vi "simple Calibration.vi"() -> ()   [LabVIEW 2020]
uses:
  <vilib>/vision/NI_Vision_Development_Module.lvlib
panel:
  out "Number of Particles":i32
  in  "stop":bool
  out "Image":T1(plugin-control)
  out "error out":errorcluster
  out "Distanza punto iniziale-finale [mm]":sgl[](array[numeric]) format="%.2f"
  in  "P1":i32
  in  "P0":i32
  in  "error in":errorcluster
  in  "Input Image Path":path=path "C:/Users/Dell/Desktop/Esame/LOAD/SimpleCalibration/CalibGrid2_Crop.png"
  out "Image":T1(plugin-control)
  in  "Risoluzione Spaziale":T2={"X Step"=1.0, "Y Step"=1.0, "Unit"=enum."Undefined"} {"Y Step" format="%.2f"; "X Step" format="%.2f"}
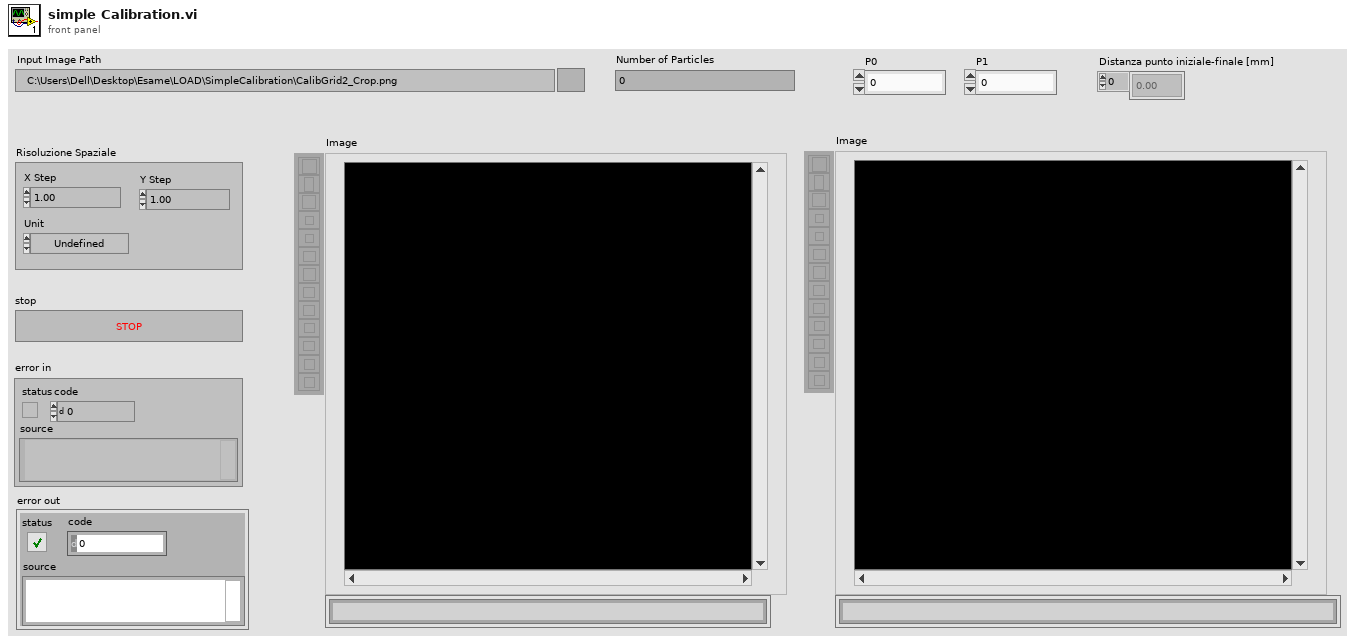
[diagram p1: front panel]
types:
  T1 = typedef "IMAQ Image.ctl" = refnum<image>
  T2 = typedef "Simple Grid Descriptor" = cluster{"X Step":sgl, "Y Step":sgl, "Unit":T3}
  T3 = typedef "Image Unit" = enum32{"Undefined", "Angström", "Micrometer", "Millimeter", "Centimeter", "Meter", "Kilometer", "Microinch", "Inch", "Feet", "Nautical miles", "Standard miles", "Steps"}
  T4 = cluster{"Area":dbl, "Number of Holes":dbl, "Bounding Rect":cluster{"Left":dbl, "Top":dbl, "Right":dbl, "Bottom":dbl}, "Center of Mass":cluster{"X":dbl, "Y":dbl}, "Orientation":dbl, "Dimensions":cluster{"Width":dbl, "Height":dbl}}[]
  T5 = cluster{"Desired Font (Application)":enum16{"User-specified Font", "Application Font", "System Font", "Dialog Font"}, "[User-specified Font]":cluster{"Font Name":string, "Size":i16, "Strikeout?":bool, "Italic?":bool, "Underline?":bool, "Outline?":bool, "Shadow?":bool, "Bold?":bool, "Rotation Angle":dbl}, "Horizontal Alignment":i16, "Vertical Alignment":i16}
  T6 = cluster{"Left":dbl, "Top":dbl, "Right":dbl, "Bottom":dbl}
  T7 = cluster{"Area":dbl, "Number of Holes":dbl, "Bounding Rect":cluster{"Left":dbl, "Top":dbl, "Right":dbl, "Bottom":dbl}, "Center of Mass":cluster{"X":dbl, "Y":dbl}, "Orientation":dbl, "Dimensions":cluster{"Width":dbl, "Height":dbl}}
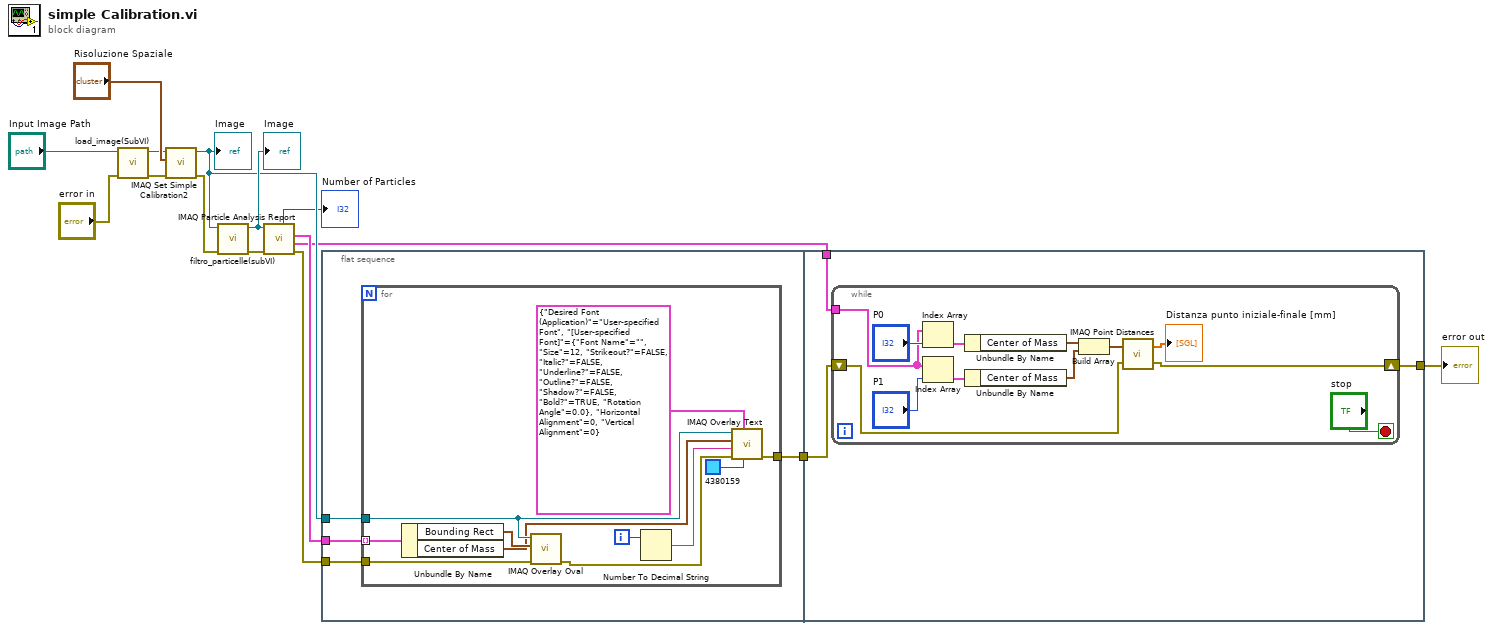
[diagram p0: block diagram]
diagram:
  n1 = call "load_image(SubVI).vi"("error in (no error)"="error in", "Image Path"="Input Image Path") -> ("error out"=w11:errorcluster, "Image GRAY"=w12:T1)  [unwired: 8 in]
  n2 = call "IMAQ Set Simple Calibration2"("error in (no error)"=w11, "Pixel Distances"="Risoluzione Spaziale", "Image"=w12) -> ("error out"=w10:errorcluster, "Calibration Template Image"=w6:T1)  [unwired: 7 in]
  "Image" <- w6
  n3 = call "filtro_particelle(subVI).vi"("error in (no error)"=w10, "Image Src"=w6) -> ("error out"=w8:errorcluster, "Image"=w9:T1)  [unwired: 8 in]
  "Image" <- w9
  n4 = call "IMAQ Particle Analysis Report"("error in (no error)"=w8, "Image"=w9) -> ("error out"=w7:errorcluster, "Particle Reports (Real-World)"=w2:T4, "Particle Reports (Pixels)"=w5:T4, "Number of Particles"=→"Number of Particles":i32)  [unwired: 4 in, 2 out]
  n5 = flat-sequence {
    tunnel: w7 -> [w19]
    tunnel: w6 -> [w18]
    tunnel: w5 -> [w17]
    tunnel: [w16] -> w3
    tunnel: [w33] -> w4
    tunnel: w3 -> [w32]
    tunnel: w2 -> [w31]
    frame #0 {
      n6 = for {
        tunnel: w19 -> [w30]
        tunnel: w18 -> [w27]
        tunnel: w17 -> [w29] mode=indexing
        tunnel: [w24] -> w16
        i -> [w23]
        n7 = Unbundle By Name(w29) -> ("Bounding Rect"=w28:T6, "Center of Mass"=w26:cluster{"X":dbl, "Y":dbl})
        n8 = call "IMAQ Overlay Oval"("error in (no error)"=w30, "Bounding Rectangle"=w28, "Image"=w27) -> ("error out"=w25:errorcluster)  [unwired: 7 in, 1 out]
        n9 = Number To Decimal String(number=w23) -> (decimal integer string=w22:string)  [unwired: 1 in]
        n10 = call "IMAQ Overlay Text"("Text Color (black)"=u32 4380159, "Font, Size & Style"=T5 {"Desired Font (Application)"=enum."User-specified Font", "[User-specified Font]"={"Font Name"="", "Size"=12, "Strikeout?"=FALSE, "Italic?"=FALSE, "Underline?"=FALSE, "Outline?"=FALSE, "Shadow?"=FALSE, "Bold?"=TRUE, "Rotation Angle"=0.0}, "Horizontal Alignment"=0, "Vertical Alignment"=0}, "error in (no error)"=w25, "String"=w22, "Origin"=w26, "Image"=w27) -> ("error out"=w24:errorcluster)  [unwired: 4 in, 1 out]
      }
    }
    frame #1 {
      n11 = while {
        tunnel: w31 -> [w34]
        shift-right: [w37] -> w33
        shift-left: w32 -> [w38]
        stop <- "stop" stop-if-true
        n12 = Index Array(array=w34, index="P0") -> (element=w45:T7)
        n13 = Index Array(array=w34, index="P1") -> (element=w42:T7)
        n14 = Unbundle By Name(w45) -> ("Center of Mass"=w40:cluster{"X":dbl, "Y":dbl})
        n15 = Unbundle By Name(w42) -> ("Center of Mass"=w41:cluster{"X":dbl, "Y":dbl})
        n16 = Build Array(w40, w41) -> (w39:cluster{"X":dbl, "Y":dbl}[])
        n17 = call "IMAQ Point Distances"("Points"=w39, "error in (no error)"=w38) -> ("Distances"=→"Distanza punto iniziale-finale [mm]":sgl[], "error out"=w37:errorcluster)  [unwired: 3 in]
      }
    }
  }
  "error out" <- w4
